vi "Critical.vi"(7 "Message":string, 8 "error in (no error)":errorcluster, 11 "Logger in":refnum<class "Logger.lvclass">) -> (0 "error out":errorcluster, 3 "Logger out":refnum<class "Logger.lvclass">)   [LabVIEW 2022 SP3, in "Logger.lvlib" / "Logger.lvclass"]
uses:
  Logger.lvclass
  C:/Users/jakub/repos/gh/sw4sys/lv-logger/PythonWrapper/Source/PythonSession/PythonSession.lvclass
  C:/Users/jakub/repos/gh/sw4sys/lv-logger/PythonWrapper/Source/PythonWrapper/PythonWrapper.lvclass
  C:/Users/jakub/repos/gh/sw4sys/lv-logger/Logger/Source/LoggingWrapper/LoggingWrapper.lvclass
  PythonWrapper/Source/PythonSession/PythonSession.lvclass/PythonSession.ctl
  PythonWrapper/Source/PythonWrapper/PythonWrapper.lvclass/PythonWrapper.ctl
  LoggingWrapper/LoggingWrapper.lvclass/LoggingWrapper.ctl
  Logger.lvclass/Logger.ctl
  PythonWrapper/Source/PythonSession/Read PythonSession.vi
  PythonWrapper/Source/PythonWrapper/Read ModulePath.vi
  Read Name.vi
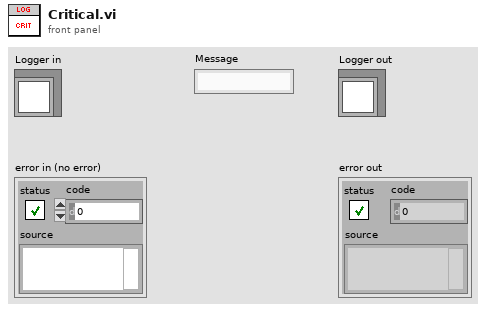
[diagram p1: front panel]
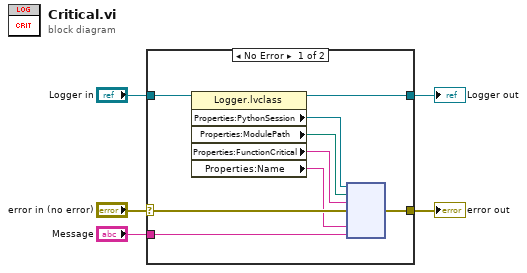
[diagram p0: block diagram]
diagram:
  n1 = case shown="No Error" "error in (no error)" {
    selector: "error in (no error)" -> [w12 w16]
    tunnel: [w11 w16] -> w1
    tunnel: [w13 w15] -> w3
    tunnel: "Logger in" -> [w14 w15]
    tunnel: "Message" -> [w7 _]
    frame No Error {
      n2 = property class="Logger.lvclass"(reference=w14) -> (reference out=w13:refnum<class "Logger.lvclass">, "Properties:PythonSession"=w10:refnum<k35>, "Properties:ModulePath"=w8:path, "Properties:FunctionCritical"=w9:string, "Properties:Name"=w6:string)  [unwired: 1 in, 1 out]
      n3 = node(w10, w8, w9, w12, w6, w7) -> (w11:errorcluster)  [unwired: 4 in, 3 out]
    }
    frame Error {
    }
  }
  "error out" <- w1
  "Logger out" <- w3
